vi "Collect UI Refs.vi"(7 "VI Refnum":refnum<vi>, 10 "Container":refnum<vi>) -> (3 "UI Refs":T1)   [LabVIEW 2020, in "OOPanel.lvlib" / "ArrayManager.lvclass"]
uses:
  ArrayManager.lvclass
  UI Refs.ctl
panel:
  out "error out":errorcluster
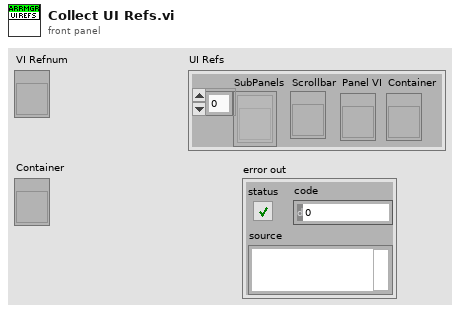
[diagram p1: front panel]
types:
  T1 = typedef "OOPanel.lvlib/ArrayManager.lvclass/UI Refs.ctl" = cluster{"SubPanels":refnum<vi>[], "Scrollbar":refnum<vi>, "Panel VI":refnum<vi>, "Container":refnum<vi>}
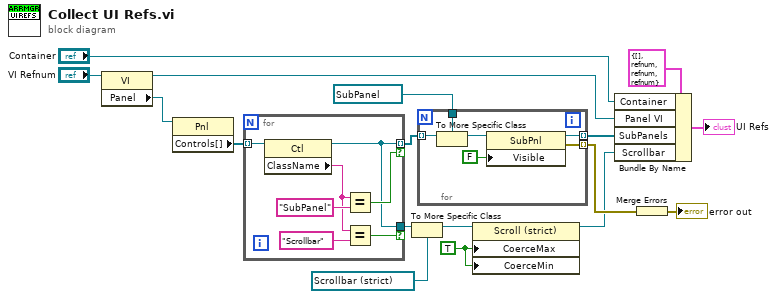
[diagram p0: block diagram]
diagram:
  w2 = TRUE ("Coerce Maximum Value")
  n1 = property on="Property Node" class="VI"(reference="VI Refnum") -> (reference out=w8:refnum<vi>, "Panel"=w12:refnum<vi>)  [unwired: 1 in, 1 out]
  n2 = property on="Property Node" class="Pnl"(reference=w12) -> ("Controls[]"=w17:refnum<vi>[])  [unwired: 1 in, 2 out]
  n3 = for {
    tunnel: w17 -> [w24] mode=indexing
    tunnel: [w19] -> w15 mode=indexing if=w22
    tunnel: [w19] -> w13 if=w18
    n4 = property class="Ctl"(reference=w24) -> (reference out=w19:refnum<vi>, "ClassName"=w21:string)  [unwired: 1 in, 1 out]
    n5 = Equal?(x=w21, y="SubPanel") -> (x = y?=w22:bool)
    n6 = Equal?(x=w21, y="Scrollbar") -> (x = y?=w18:bool)
  }
  n7 = To More Specific Class(target class=refnum<vi> refnum ("Scrollbar"), reference=w13) -> (specific class reference=w3:refnum<vi>)  [unwired: 1 in, 1 out]
  n8 = for {
    tunnel: w15 -> [w30] mode=indexing
    tunnel: [w26] -> w9 mode=indexing
    tunnel: refnum<vi> refnum ("target class") -> [w29]
    tunnel: [w25] -> w5 mode=indexing
    n9 = To More Specific Class(target class=w29, reference=w30) -> (specific class reference=w28:refnum<vi>)  [unwired: 1 in, 1 out]
    n10 = property class="SubPnl"(reference=w28, "Visible"=FALSE) -> (reference out=w26:refnum<vi>, error out=w25:errorcluster)  [unwired: 1 in]
  }
  n11 = property class="Scroll (strict)"(reference=w3, "CoerceMax"=w2, "CoerceMin"=w2) -> (reference out=w1:refnum<vi>)  [unwired: 1 in, 1 out]
  n12 = Bundle By Name(cluster=T1 {"SubPanels"=[], "Scrollbar"=refnum, "Panel VI"=refnum, "Container"=refnum} ("UI Refs"), "Container"="Container", "Panel VI"=w8, "SubPanels"=w9, "Scrollbar"=w1) -> (→"UI Refs":T1)
  n13 = Merge Errors(w5) -> (→"error out":errorcluster)
